vi "KlingerV2 VisaRW.vi"(0 "VISA Rsrc":refnum<visa-resource-name>="SR530", 2 "EOS (Aucun)":string, 3 "Délais (0 ms)":u32, 5 "ChaineCom":string caption="Chaîne de commande", 7 "Nbcomm":i32=1 caption="Nombre de \nCommandes", 9 "Nbcaract":u32=100 caption="Nombre de \ncaractères à lire", 11 "error in (no error)":errorcluster, 12 "Lecture?(T)":bool=TRUE, 13 "Poll?(F)":bool) -> (4 "VISA Rsrc Out":refnum<visa-resource-name>="GPIB0::12::INSTR", 6 "ChaineRep":string caption="Chaîne de réponse", 8 "octet d'état":u16, 14 "Count out":u32=44 caption="Nombre de caractères lus", 15 "error out":errorcluster)   [LabVIEW 2010]
doc: "Ce VI envoie des commande d'écriture et de lecture VISA à l'appareil GPIB. Il permet de ne pas séparer un question de sa réponse. Pour que cela fonctionne toute lecture d'un instrument doit se faire par ce VI."
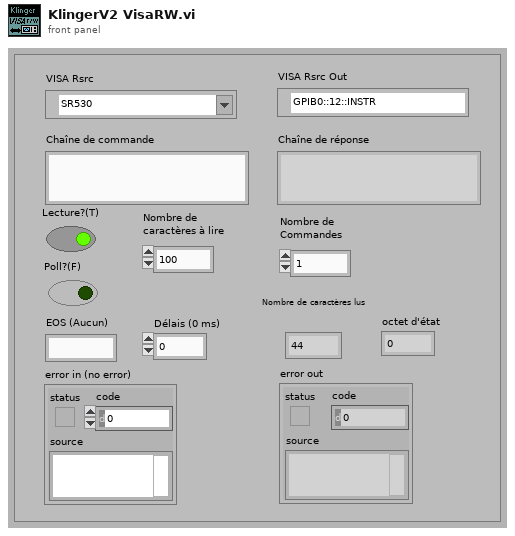
[diagram p1: front panel]
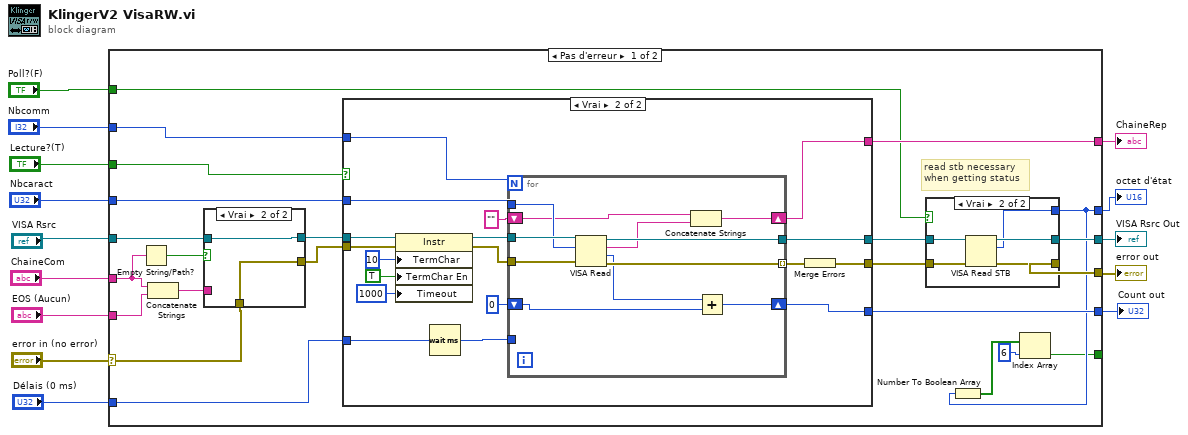
[diagram p0: block diagram]
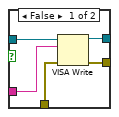
[diagram p3: hidden frame]
diagram:
  n1 = case shown="Pas d'erreur" "error in (no error)" {
    selector: "error in (no error)" -> [w34 w84]
    tunnel: "VISA Rsrc" -> [w35 w83]
    tunnel: [w20 w83] -> w7
    tunnel: "ChaineCom" -> [w25 _]
    tunnel: "EOS (Aucun)" -> [w37 _]
    tunnel: "Délais (0 ms)" -> [w31 _]
    tunnel: "Nbcaract" -> [w30 _]
    tunnel: "Lecture?(T)" -> [w29 _]
    tunnel: [w19 w84] -> w9
    tunnel: "Nbcomm" -> [w26 _]
    tunnel: [w28 _] -> w5
    tunnel: [w27 _] -> w4
    tunnel: "Poll?(F)" -> [w23 _]
    tunnel: [w16 _] -> w1
    tunnel: [w15 _] -> _
    frame No Error {
      # "read stb necessary\nwhen getting status"
      n2 = Empty String/Path?(string/path=w25) -> (empty?=w24:bool)
      n3 = Concatenate Strings(w25, w37) -> (w36:string)
      n4 = case shown="Vrai" w24 {
        tunnel: w36 -> [w49 _]
        tunnel: w35 -> [w48 w51]
        tunnel: w34 -> [w47 w50]
        tunnel: [w46 w51] -> w33
        tunnel: [w45 w50] -> w32
        frame False {
          n5 = VISA Write(VISA resource name=w48, write buffer=w49, error in (no error)=w47) -> (VISA resource name out=w46:refnum<visa-resource-name>, error out=w45:errorcluster)  [unwired: 1 out]
        }
        frame True {
        }
      }
      n6 = case shown="Vrai" w29 {
        tunnel: w33 -> [w53 w71]
        tunnel: [w53 w55] -> w21
        tunnel: w32 -> [w52 w60]
        tunnel: [w52 w54] -> w22
        tunnel: w30 -> [_ w69]
        tunnel: w31 -> [_ w68]
        tunnel: w26 -> [_ w62]
        tunnel: [_ w64] -> w28
        tunnel: [_ w63] -> w27
        frame False {
        }
        frame True {
          n7 = property class="Instr"(reference=w71, error in=w60, "TermChar"=u8 10 ("Message Based Settings:Termination Character"), "TermChar En"=TRUE ("Message Based Settings:Termination Character Enable"), "Timeout"=u32 1000 ("General Settings:Timeout Value")) -> (reference out=w61:refnum<visa-resource-name>, error out=w59:errorcluster)
          n8 = Wait (ms)(milliseconds to wait=w68) -> (millisecond timer value=w67:u32)
          n9 = for {
            N: w62 -> [_]
            tunnel: w61 -> [w82]
            tunnel: [w81] -> w55
            tunnel: w59 -> [w80]
            tunnel: [w79] -> w70 mode=indexing
            tunnel: w69 -> [w78]
            tunnel: w67 -> [_]
            shift-right: [w76] -> w64
            shift-left: "" -> [w75]
            shift-right: [w73] -> w63
            shift-left: u32 0 -> [w72]
            n10 = VISA Read(VISA resource name=w82, byte count=w78, error in (no error)=w80) -> (VISA resource name out=w81:refnum<visa-resource-name>, read buffer=w77:string, return count=w74:u32, error out=w79:errorcluster)
            n11 = Concatenate Strings(w75, w77) -> (w76:string)
            n12 = Add(x=w74, y=w72) -> (x+y=w73:u32)
          }
          n13 = Merge Errors(w70) -> (w54:errorcluster)
        }
      }
      n14 = case shown="Vrai" w23 {
        tunnel: [w39 w44] -> w20
        tunnel: [w38 w43] -> w19
        tunnel: w22 -> [w38 w42]
        tunnel: w21 -> [w39 w41]
        tunnel: [_ w40] -> w16
        frame False {
        }
        frame True {
          n15 = VISA Read STB(8:w42, 11:w41) -> (0:w43:errorcluster, 2:w40:u16, 3:w44:refnum<visa-resource-name>)
        }
      }
      n16 = Number To Boolean Array(number=w16) -> (Boolean array=w17:bool[])
      n17 = Index Array(array=w17, index=6) -> (element=w15:bool)
    }
    frame Error {
    }
  }
  "error out" <- w9
  "VISA Rsrc Out" <- w7
  "ChaineRep" <- w5
  "Count out" <- w4
  "octet d'état" <- w1
